vi "Searchable Tag.vi"(11 "SectionProperties":T1) -> (3 "Section data entry for file":string)   [LabVIEW 2019, in "DataLog.lvclass"]
doc: "Use this in the datalogger for generating a file section, and for generating a seciton to search for"
uses:
  DataLog.lvclass
  SearchableTag.ctl
  Sequence/SequenceSubvis/RF Direction.ctl
  Sequence/SequenceSubvis/PolarizationSelect.ctl
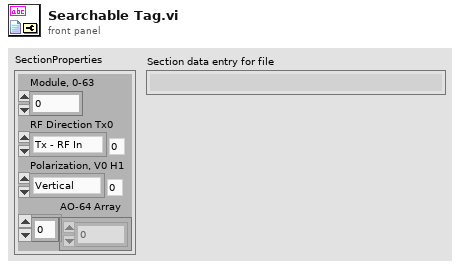
[diagram p1: front panel]
types:
  T1 = typedef "DataLog.lvclass/SearchableTag.ctl" = cluster{"Module, 0-63":i32, "RF Direction Tx0":T2, "Polarization, V0 H1":T3, "AO-64 Array":dbl[]}
  T2 = typedef "RF Direction.ctl" = enum16{"Tx - RF In", "Rx - RF Out"}
  T3 = typedef "PolarizationSelect.ctl" = enum16{"Vertical", "Horizontal"}
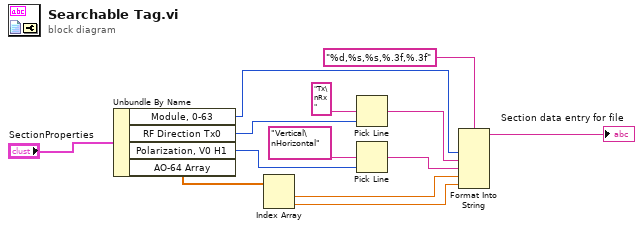
[diagram p0: block diagram]
diagram:
  n1 = Unbundle By Name("SectionProperties") -> ("Module, 0-63"=w7:i32, "RF Direction Tx0"=w6:T2, "Polarization, V0 H1"=w11:T3, "AO-64 Array"=w3:dbl[])
  n2 = Index Array(array=w3) -> (element #1=w2:dbl, element #2=w1:dbl)  [unwired: 2 in]
  n3 = Pick Line(multi-line string="Tx\nRx", line index=w6) -> (output string=w4:string)  [unwired: 1 in]
  n4 = Pick Line(multi-line string="Vertical\nHorizontal", line index=w11) -> (output string=w5:string)  [unwired: 1 in]
  n5 = Format Into String(format string="%d,%s,%s,%.3f,%.3f", w7, w4, w5, w2, w1) -> (resulting string=→"Section data entry for file":string)  [unwired: 2 in, 1 out]
